vi "DG635 Set Pulse Timing.vi"(7 "Output pulse channel":T1, 8 "error in":errorcluster, 9 "Duration":dbl format="%#_6ps", 10 "Start delay":dbl format="%#_6ps", 11 "VISA resource name":refnum<visa-resource-name>) -> (0 "error out":errorcluster, 2 "Status byte":i32 format="%b", 3 "VISA resource name out":refnum<visa-resource-name>)   [LabVIEW 2020]
uses:
  DG Pulse Output Channel.ctl
  DG635 Channel.ctl
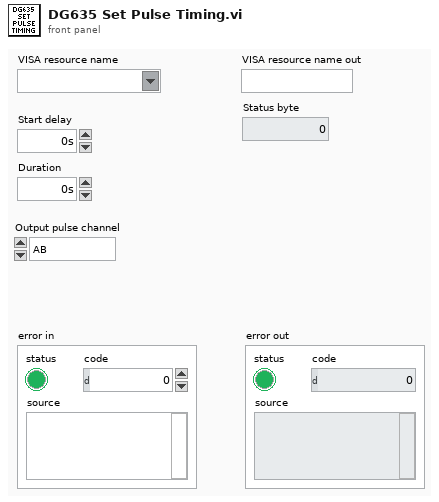
[diagram p1: front panel]
types:
  T1 = typedef "DG Pulse Output Channel.ctl" = enum16{"AB", "CD"}
  T2 = typedef "DG635 Channel.ctl" = enum16{"T0", "T1", "A", "B", "C", "D", "E", "F", "G", "H"}
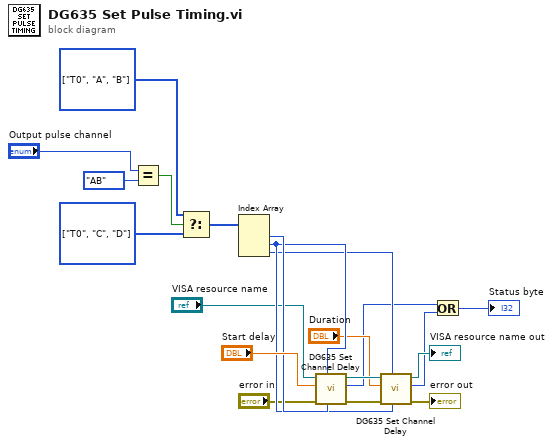
[diagram p0: block diagram]
diagram:
  w17 = T2[] [enum."T0", enum."C", enum."D"] items=["T0", "T1", "A", "B", "C", "D", "E", "F", "G", "H"]
  w18 = T2[] [enum."T0", enum."A", enum."B"] items=["T0", "T1", "A", "B", "C", "D", "E", "F", "G", "H"]
  n1 = Equal?(x="Output pulse channel", y=DG_Pulse_Output_Channel."AB") -> (x = y?=w16:bool)
  n2 = Select(t=w18, s=w16, f=w17) -> (s? t:f=w14:T2[])
  n3 = Index Array(array=w14) -> (element #1=w13:T2, element #2=w12:T2, element #3=w11:T2)  [unwired: 3 in]
  n4 = call "DG635 Set Channel Delay.vi"("Relative to channel"=w13, "Output channel"=w12, "error in"="error in", "Start delay"="Start delay", "VISA resource name"="VISA resource name") -> ("error out"=w10:errorcluster, "Status byte"=w3:i32, "VISA resource name out"=w7:refnum<visa-resource-name>)  [unwired: 4 in]
  n5 = call "DG635 Set Channel Delay.vi"("Relative to channel"=w12, "Output channel"=w11, "error in"=w10, "Start delay"="Duration", "VISA resource name"=w7) -> ("error out"=→"error out":errorcluster, "Status byte"=w2:i32, "VISA resource name out"=→"VISA resource name out":refnum<visa-resource-name>)  [unwired: 4 in]
  n6 = Or(x=w3, y=w2) -> (x .or. y?=→"Status byte":i32)
